vi "3_3.vi"() -> ()   [LabVIEW 2019]
panel:
  in  "stop":bool
  out "Waveform Chart":dynamicdata(graph)
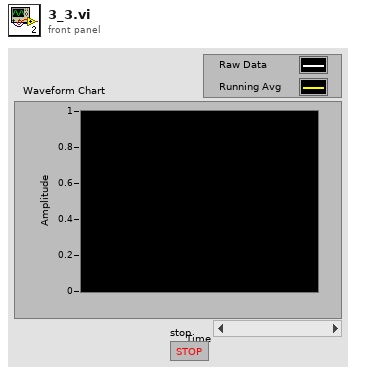
[diagram p1: front panel]
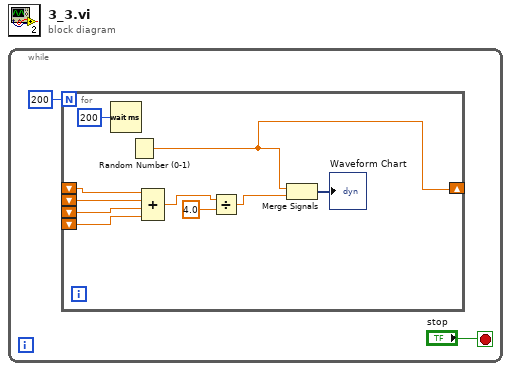
[diagram p0: block diagram]
diagram:
  n1 = while {
    stop <- "stop" stop-if-true
    n2 = for {
      N: 200 -> [_]
      shift-right: [w5] -> _
      shift-left: _ -> [w12]
      shift-left: _ -> [w11]
      shift-left: _ -> [w10]
      shift-left: _ -> [w9]
      n3 = Wait (ms)(milliseconds to wait=u32 200) -> ()  [unwired: 1 out]
      n4 = Random Number (0-1)() -> (number: 0 to 1=w5:dbl)
      n5 = Compound Arithmetic op=ADD(w12, w11, w10, w9) -> (w7:dbl)
      n6 = Divide(x=w7, y=4.0) -> (x/y=w4:dbl)
      n7 = Merge Signals(w5, w4) -> (→"Waveform Chart":dynamicdata)
    }
  }
